vi "Manual Test - New Type Def.vi"() -> ()   [LabVIEW 2020]
panel:
  out "Error Out":errorcluster
  in  "Cluster Name":string="Blah"
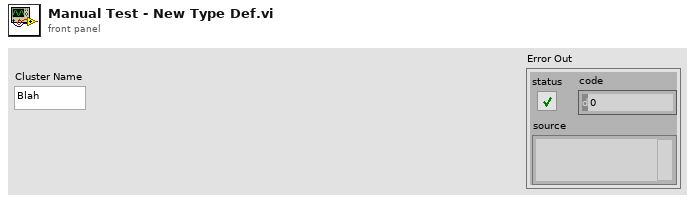
[diagram p1: front panel]
types:
  T1 = enum32{"invalid VI type", "Standard VI", "Control VI", "Global VI", "Polymorphic VI", "Configuration VI", "SubSystem", "Facade VI", "Method VI", "Statechart Diagram VI"}
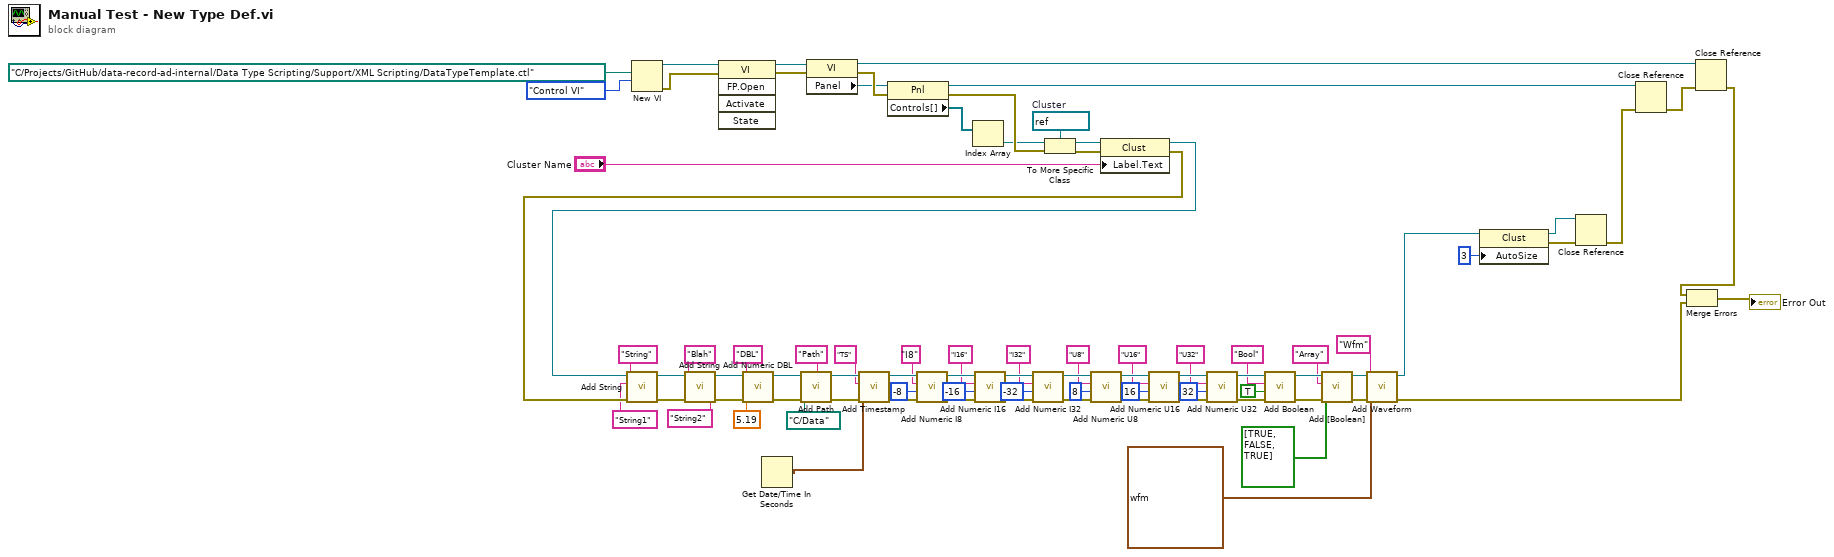
[diagram p0: block diagram]
diagram:
  w68 = refnum<vi> refnum  # Cluster
  n1 = New VI(9:T1."Control VI" ("vi type (standard vi)"), 10:path "C:/Projects/GitHub/data-record-ad-internal/Data Type Scripting/Support/XML Scripting/DataTypeTemplate.ctl" ("template")) -> (0:w77:errorcluster, 3:w78:refnum<vi>)  [unwired: 5 in]
  n2 = invoke class="VI" method="FP.Open"(reference=w78, error in=w77) -> (reference out=w76:refnum<vi>, error out=w69:errorcluster)  [unwired: 3 in, 3 out]
  n3 = Get Date/Time In Seconds() -> (seconds since 1Jan1904=w23:timestamp)
  n4 = property class="VI"(reference=w76, error in=w69) -> (reference out=w11:refnum<vi>, error out=w81:errorcluster, "Panel"=w75:refnum<vi>)
  n5 = property class="Pnl"(reference=w75, error in=w81) -> (reference out=w12:refnum<vi>, error out=w82:errorcluster, "Controls[]"=w74:refnum<vi>[])
  n6 = Index Array(array=w74) -> (element=w72:refnum<vi>)  [unwired: 1 in]
  n7 = To More Specific Class(target class=w68, reference=w72, error in=w82) -> (specific class reference=w71:refnum<vi>, error out=w70:errorcluster)
  n8 = property class="Clust"(reference=w71, error in=w70, "Label.Text"="Cluster Name") -> (reference out=w66:refnum<vi>, error out=w67:errorcluster)
  n9 = call "Add String.vi"("error in (no error)"=w67, "Value"="String", "Label Text"="String1" ("Label.Text"), "Cluster in"=w66) -> ("error out"=w59:errorcluster, "Cluster out"=w60:refnum<vi>)  [unwired: 6 in]
  n10 = call "Add String.vi"("error in (no error)"=w59, "Value"="Blah", "Label Text"="String2" ("Label.Text"), "Cluster in"=w60) -> ("error out"=w58:errorcluster, "Cluster out"=w57:refnum<vi>)  [unwired: 6 in]
  n11 = call "Add Numeric DBL.vi"("error in (no error)"=w58, "Value"=5.19, "Label Text"="DBL" ("Label.Text"), "Cluster in"=w57) -> ("error out"=w54:errorcluster, "Cluster out"=w53:refnum<vi>)  [unwired: 6 in]
  n12 = call "Add Path.vi"("error in (no error)"=w54, "Value"=path "C:/Data", "Label Text"="Path", "Cluster in"=w53) -> ("error out"=w50:errorcluster, "Cluster out"=w47:refnum<vi>)  [unwired: 6 in]
  n13 = call "Add Timestamp.vi"("error in (no error)"=w50, "Value"=w23, "Label Text"="TS", "Cluster in"=w47) -> ("error out"=w49:errorcluster, "Cluster out"=w46:refnum<vi>)  [unwired: 6 in]
  n14 = call "Add Numeric I8.vi"("error in (no error)"=w49, "Value"=i8 -8, "Label Text"="I8", "Cluster in"=w46) -> ("error out"=w48:errorcluster, "Cluster out"=w45:refnum<vi>)  [unwired: 6 in]
  n15 = call "Add Numeric I16.vi"("error in (no error)"=w48, "Value"=i16 -16, "Label Text"="I16", "Cluster in"=w45) -> ("error out"=w43:errorcluster, "Cluster out"=w44:refnum<vi>)  [unwired: 6 in]
  n16 = call "Add Numeric I32.vi"("error in (no error)"=w43, "Value"=-32, "Label Text"="I32", "Cluster in"=w44) -> ("error out"=w41:errorcluster, "Cluster out"=w42:refnum<vi>)  [unwired: 6 in]
  n17 = call "Add Numeric U8.vi"("error in (no error)"=w41, "Value"=u8 8, "Label Text"="U8", "Cluster in"=w42) -> ("error out"=w39:errorcluster, "Cluster out"=w40:refnum<vi>)  [unwired: 6 in]
  n18 = call "Add Numeric U16.vi"("error in (no error)"=w39, "Value"=u16 16, "Label Text"="U16", "Cluster in"=w40) -> ("error out"=w37:errorcluster, "Cluster out"=w38:refnum<vi>)  [unwired: 6 in]
  n19 = call "Add Numeric U32.vi"("error in (no error)"=w37, "Value"=u32 32, "Label Text"="U32", "Cluster in"=w38) -> ("error out"=w35:errorcluster, "Cluster out"=w36:refnum<vi>)  [unwired: 6 in]
  n20 = call "Add Boolean.vi"("error in (no error)"=w35, "Value"=TRUE, "Label Text"="Bool", "Cluster in"=w36) -> ("error out"=w29:errorcluster, "Cluster out"=w28:refnum<vi>)  [unwired: 6 in]
  n21 = call "Add [Boolean].vi"("error in (no error)"=w29, "Value"=bool[] [TRUE, FALSE, TRUE], "Label Text"="Array", "Cluster in"=w28) -> ("error out"=w8:errorcluster, "Cluster out"=w7:refnum<vi>)  [unwired: 6 in]
  n22 = call "Add Waveform.vi"("error in (no error)"=w8, "Value"=waveform(dbl) {"t0"=timestamp(0 s since 1904-01-01), "dt"=1.0, "Y"=[]}, "Label Text"="Wfm", "Cluster in"=w7) -> ("error out"=w2:errorcluster, "Cluster out"=w6:refnum<vi>)  [unwired: 6 in]
  n23 = property class="Clust"(reference=w6, "AutoSize"=u32 3 ("Auto Sizing")) -> (reference out=w13:refnum<vi>, error out=w14:errorcluster)  [unwired: 1 in]
  n24 = Close Reference(reference=w13, error in (no error)=w14) -> (error out=w10:errorcluster)
  n25 = Close Reference(reference=w12, error in (no error)=w10) -> (error out=w9:errorcluster)
  n26 = Close Reference(reference=w11, error in (no error)=w9) -> (error out=w3:errorcluster)
  n27 = Merge Errors(w3, w2) -> (→"Error Out":errorcluster)
